vi "Collect All Positions.vi"(0 "Input [tag_id, anchor_id, distance, time]":string[][](array[string]), 1 "Anchor 2 Y":dbl, 2 "Anchor 1 X":dbl, 3 "Anchor 1 Y":dbl, 4 "Anchor 3 X":dbl, 5 "Anchor 2 X":dbl, 6 "Anchor 3 Y":dbl) -> (7 "Positions":cluster{"X":dbl, "Y":dbl}[](array[cluster]), 8 "Positions + distance batch":T1(array[cluster]))   [LabVIEW 2014]
uses:
  Position.lvclass
panel:
  out "Positions array":dbl[][](array[numeric])
  out "y2 3":dbl
  out "x2 3":dbl
  out "y1 3":dbl
  out "x1 3":dbl
  out "y2 2":dbl
  out "x2 2":dbl
  out "y1 2":dbl
  out "x1 2":dbl
  out "y2 1":dbl
  out "x2 1":dbl
  out "y1 1":dbl
  out "x1 1":dbl
  out "R anch 3":dbl
  out "R anch 2":dbl
  out "R anch 1":dbl
  in  "Intersections":T2(array[cluster])
  # "All anchor x, y coordinates"
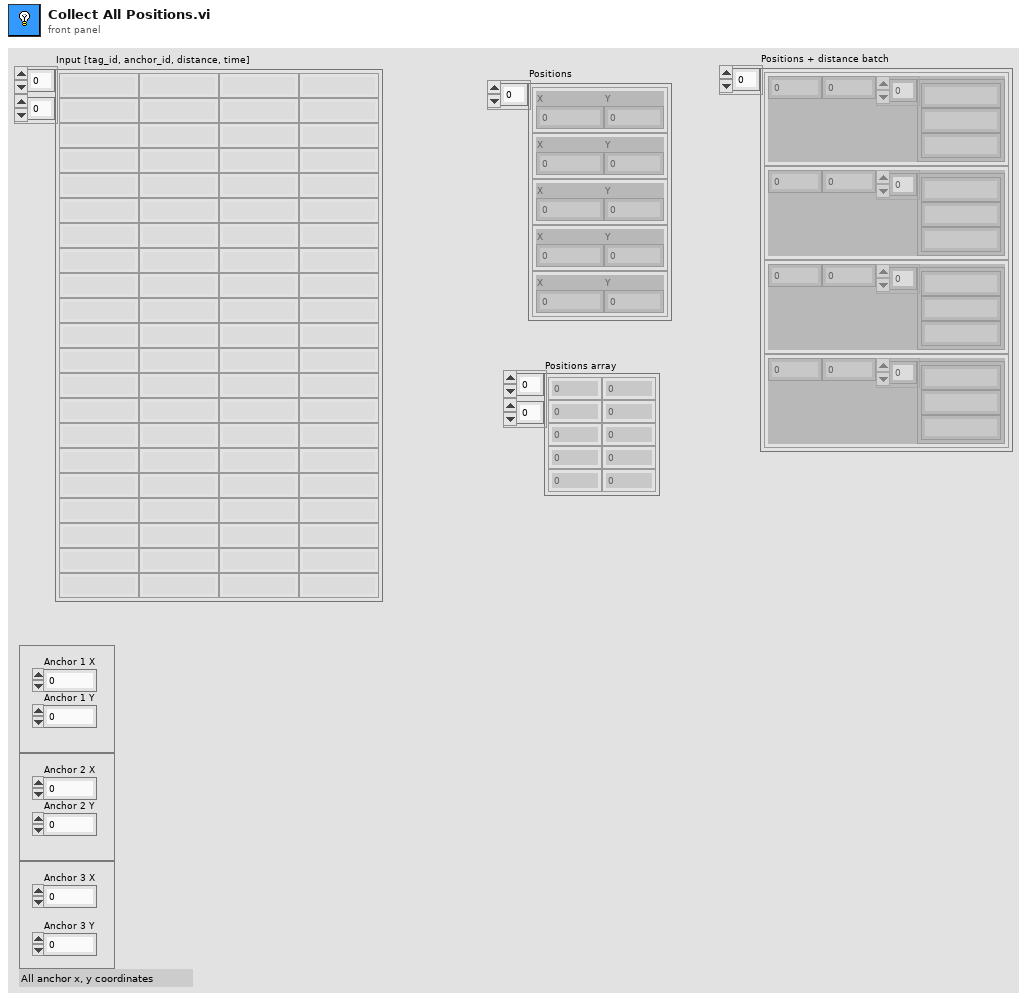
[diagram p1: front panel]
types:
  T1 = cluster{"X":dbl, "Y":dbl, "Batch array":string[]}[]
  T2 = cluster{"time [ms]":dbl, "y":dbl, "x":dbl, "Fout":bool, "Goed":bool}[]
  T3 = cluster{"Time [ms]":dbl, "y":dbl, "x":dbl, "Fout":bool, "Goed":bool}[]
  T4 = cluster{"Y":dbl, "X":dbl, "Batch array":string[]}
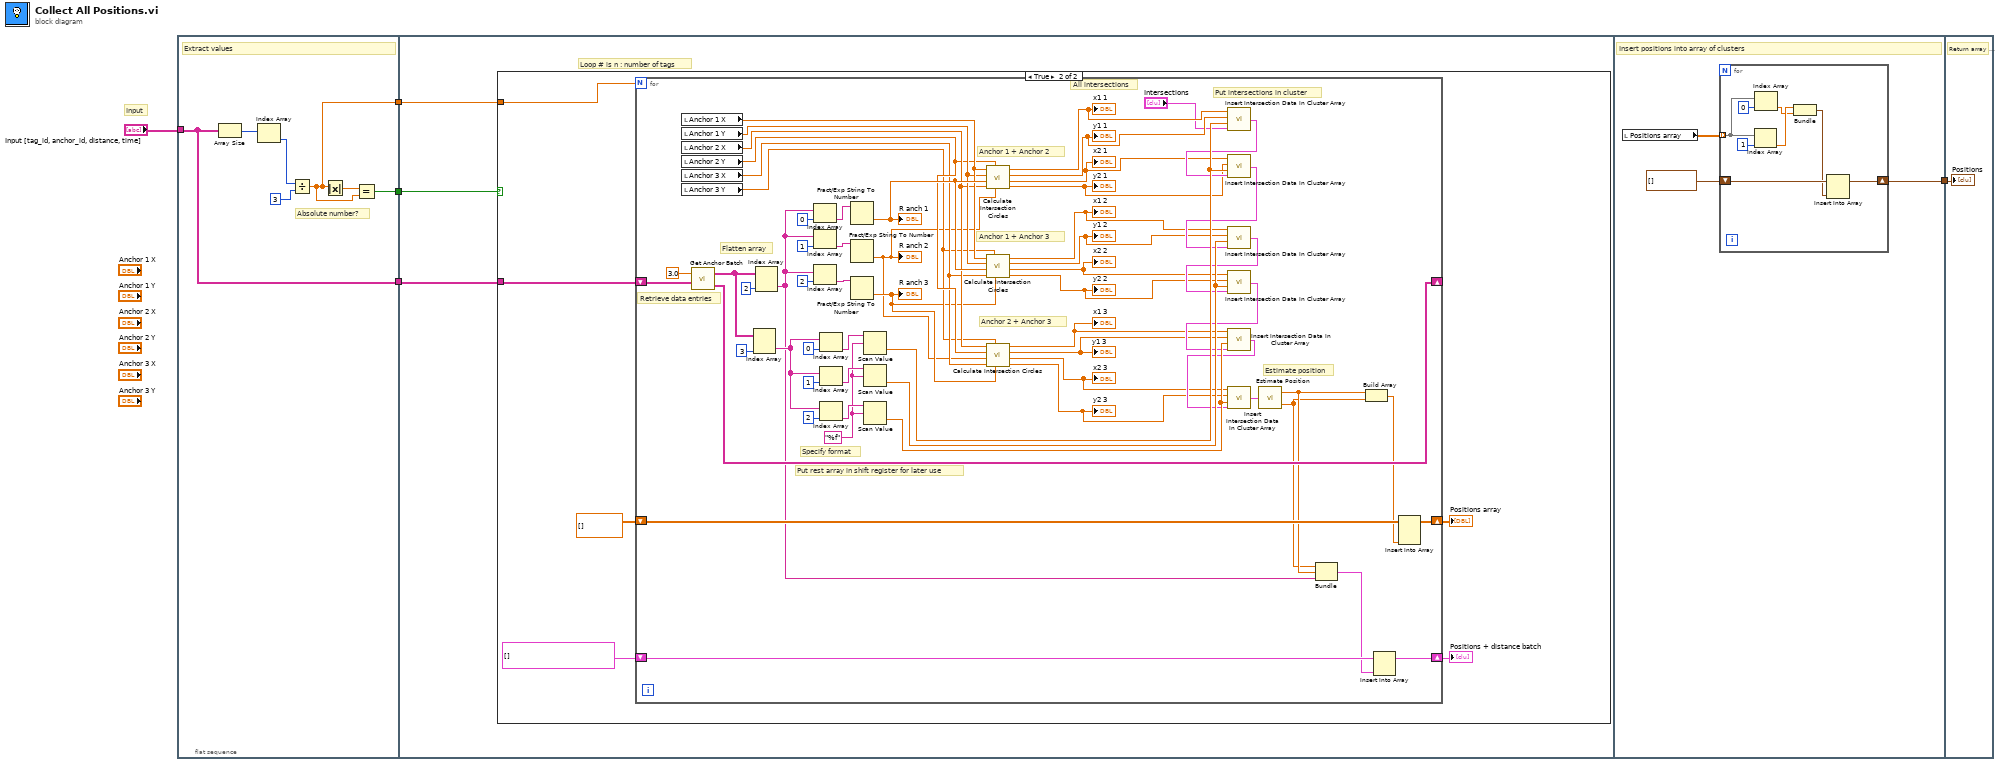
[diagram p0: block diagram]
diagram:
  # "Input"
  n1 = flat-sequence {
    tunnel: "Input [tag_id, anchor_id, distance, time]" -> [w7]
    tunnel: [w8] -> w4
    tunnel: [w7] -> w3
    tunnel: [w6] -> w2
    tunnel: w4 -> [w15]
    tunnel: w3 -> [w14]
    tunnel: w2 -> [w13]
    tunnel: [w82] -> w1
    tunnel: w1 -> [w93]
    frame #0 {
      # "Absolute number?"
      # "Extract values"
      n2 = Array Size(array=w7) -> (size(s)=w12:i32[])
      n3 = Index Array(array=w12) -> (element=w9:i32)  [unwired: 1 in]
      n4 = Divide(x=w9, y=3) -> (x/y=w6:dbl)
      n5 = Absolute Value(x=w6) -> (abs(x)=w10:dbl)
      n6 = Equal?(x=w10, y=w6) -> (x = y?=w8:bool)
    }
    frame #1 {
      # "Loop # is n : number of tags"
      n7 = case shown="True" w15 {
        tunnel: w14 -> [_ w21]
        tunnel: w13 -> [_ w20]
        frame False {
          # "Todo"
        }
        frame True {
          n8 = for {
            N: w20 -> [_]
            shift-right: [w78] -> _
            shift-left: w21 -> [w79]
            shift-right: [w30] -> w19
            shift-left: dbl[][] [] -> [w81]
            shift-right: [w27] -> w17
            shift-left: T1 [] ("Array constant") -> [w26]
            w61 = "%f" ("format string")
            # "Estimate position"
            # "Put intersections in cluster"
            # "All intersections"
            # "Anchor 2 + Anchor 3"
            # "Anchor 1 + Anchor 3"
            # "Anchor 1 + Anchor 2"
            # "Specify format"
            # "Retrieve data entries"
            # "Flatten array"
            # "Put rest array in shift register for later use"
            n9 = local read "Anchor 1 X"() -> (w59:dbl)
            n10 = local read "Anchor 1 Y"() -> (w58:dbl)
            n11 = local read "Anchor 2 X"() -> (w57:dbl)
            n12 = local read "Anchor 2 Y"() -> (w56:dbl)
            n13 = local read "Anchor 3 X"() -> (w55:dbl)
            n14 = local read "Anchor 3 Y"() -> (w54:dbl)
            n15 = call "Get Anchor Batch.vi"("Input Array"=w79, "Batch size"=3.0) -> ("Rest array"=w78:string[][], "Batch array"=w70:string[][])
            n16 = Index Array(array=w70, index (col)=3 ("disabled index (col)")) -> (element=w65:string[])  [unwired: 1 in]
            n17 = Index Array(array=w70, index (col)=2 ("index (row)")) -> (element=w25:string[])  [unwired: 1 in]
            n18 = Index Array(array=w25, index=0) -> (element=w73:string)
            n19 = Index Array(array=w25, index=1) -> (element=w72:string)
            n20 = Index Array(array=w25, index=2) -> (element=w71:string)
            n21 = Index Array(array=w65, index=0) -> (element=w64:string)
            n22 = Index Array(array=w65, index=1) -> (element=w63:string)
            n23 = Index Array(array=w65, index=2) -> (element=w62:string)
            n24 = Fract/Exp String To Number(string=w73) -> (number=w60:dbl)  [unwired: 3 in, 1 out]
            "R anch 1" <- w60
            n25 = Fract/Exp String To Number(string=w72) -> (number=w52:dbl)  [unwired: 3 in, 1 out]
            "R anch 2" <- w52
            n26 = Fract/Exp String To Number(string=w71) -> (number=w53:dbl)  [unwired: 3 in, 1 out]
            "R anch 3" <- w53
            n27 = Scan Value(string=w64, format string=w61) -> (value=w49:dbl)  [unwired: 1 in, 1 out]
            n28 = Scan Value(string=w63, format string=w61) -> (value=w48:dbl)  [unwired: 1 in, 1 out]
            n29 = Scan Value(string=w62, format string=w61) -> (value=w47:dbl)  [unwired: 1 in, 1 out]
            n30 = call "Calculate Intersection Circles.vi"("r2"=w52, "d"=w56, "c"=w57, "r1"=w60, "b"=w58, "a"=w59) -> ("y2"=w40:dbl, "x2"=w41:dbl, "y1"=w50:dbl, "x1"=w51:dbl)
            "x1 1" <- w51
            "y1 1" <- w50
            "x2 1" <- w41
            "y2 1" <- w40
            n31 = call "Calculate Intersection Circles.vi"("r2"=w53, "d"=w54, "c"=w55, "r1"=w60, "b"=w58, "a"=w59) -> ("y2"=w36:dbl, "x2"=w37:dbl, "y1"=w38:dbl, "x1"=w39:dbl)
            "x1 2" <- w39
            "y1 2" <- w38
            "x2 2" <- w37
            "y2 2" <- w36
            n32 = call "Calculate Intersection Circles.vi"("r2"=w53, "d"=w54, "c"=w55, "r1"=w52, "b"=w56, "a"=w57) -> ("y2"=w32:dbl, "x2"=w33:dbl, "y1"=w34:dbl, "x1"=w35:dbl)
            "x1 3" <- w35
            "y1 3" <- w34
            "x2 3" <- w33
            "y2 3" <- w32
            n33 = call "Insert Intersection Data In Cluster Array.vi"("ClusterArray"="Intersections", "Time"=w49, "Y"=w50, "X"=w51) -> ("Intersections"=w46:T3)
            n34 = call "Insert Intersection Data In Cluster Array.vi"("ClusterArray"=w46, "Time"=w49, "Y"=w40, "X"=w41) -> ("Intersections"=w45:T3)
            n35 = call "Insert Intersection Data In Cluster Array.vi"("ClusterArray"=w45, "Time"=w48, "Y"=w38, "X"=w39) -> ("Intersections"=w44:T3)
            n36 = call "Insert Intersection Data In Cluster Array.vi"("ClusterArray"=w44, "Time"=w48, "Y"=w36, "X"=w37) -> ("Intersections"=w43:T3)
            n37 = call "Insert Intersection Data In Cluster Array.vi"("ClusterArray"=w43, "Time"=w47, "Y"=w34, "X"=w35) -> ("Intersections"=w42:T3)
            n38 = call "Insert Intersection Data In Cluster Array.vi"("ClusterArray"=w42, "Time"=w47, "Y"=w32, "X"=w33) -> ("Intersections"=w31:T3)
            n39 = call "Estimate Position.vi"("Intersections"=w31) -> ("X"=w23:dbl, "Y"=w22:dbl)
            n40 = Bundle("Y"=w22, "X"=w23, "Batch array"=w25) -> (w24:T4)  [unwired: 1 in]
            n41 = Build Array(w23, w22) -> (w29:dbl[])
            n42 = Insert Into Array(array=w26, new element=w24) -> (w27:T1)  [unwired: 1 in]
            n43 = Insert Into Array(array=w81, new element=w29) -> (w30:dbl[][])  [unwired: 2 in]
          }
          "Positions array" <- w19
          "Positions + distance batch" <- w17
        }
      }
    }
    frame #2 {
      # "Insert positions into array of clusters"
      n44 = local read "Positions array"() -> (w84:dbl[][])
      n45 = for {
        tunnel: w84 -> [w91] mode=indexing
        shift-right: [w89] -> w82
        shift-left: cluster{"X":dbl, "Y":dbl}[] [] ("Positions 2") -> [w88]
        n46 = Index Array(array=w91, index=1) -> (element=w86:dbl)
        n47 = Index Array(array=w91, index=0) -> (element=w85:dbl)
        n48 = Bundle(w86, w85) -> (w87:cluster{dbl, dbl})  [unwired: 1 in]
        n49 = Insert Into Array(array=w88, new element=w87) -> (w89:cluster{"X":dbl, "Y":dbl}[])  [unwired: 1 in]
      }
    }
    frame #3 {
      # "Return array of cluster of positions"
      "Positions" <- w93
    }
  }
